vi "Populate Menu.vi"(8 "error in (no error)":errorcluster, 9 "Coords":T1, 10 "MenuRef":refnum<k9>, 11 "Test Executive View in":refnum<class "Test Executive View.lvclass">) -> (0 "error out":errorcluster, 2 "Discard?":bool, 3 "Test Executive View out":refnum<class "Test Executive View.lvclass">)   [LabVIEW 2019, in "Test Executive View.lvclass"]
uses:
  <vilib>/gpm_packages/@cs/Test-executive-builder/Example/Application/Test Executive View/Test Executive View/Test Executive View.lvclass
  C:/Program Files/National Instruments/LabVIEW 2019/vi.lib/gpm_packages/@cs/Test-executive-builder/Source/Test Executive Builder View/Test Executive Builder View/Test Executive Builder View.lvclass
  <vilib>/Utility/miscctls.llb/LVPoint32TypeDef.ctl
  <vilib>/gpm_packages/@cs/Test-executive-builder/Source/Test Executive Builder View/Test Executive Builder View/Test Executive Builder View.lvclass/Test Executive Builder View.ctl
  <vilib>/gpm_packages/@cs/Test-executive-builder/Source/Test Executive Builder View/Tree Click Interpreter/Tree Click Interpreter.lvclass
  <vilib>/gpm_packages/@cs/Test-executive-builder/Source/Test Executive Builder View/Test Executive Builder View/Test Executive Builder View.lvclass
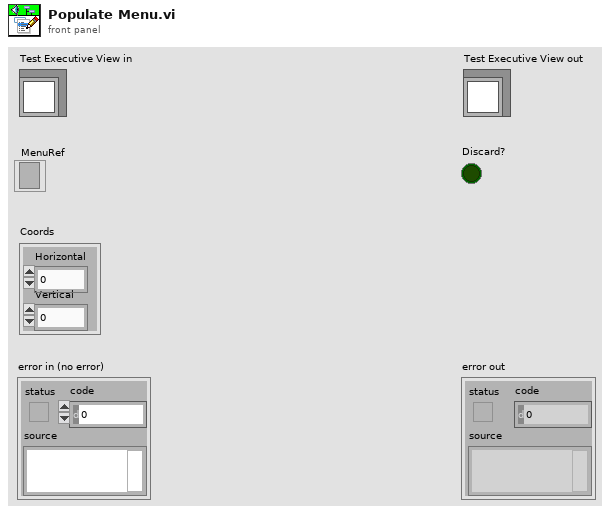
[diagram p1: front panel]
types:
  T1 = typedef "LVPoint32TypeDef.ctl" = cluster{"Horizontal":i32, "Vertical":i32}
  T2 = typedef "Relative Click Location.ctl" = enum16{"Unknown Location", "Below Element", "On Element", "Above Element"}
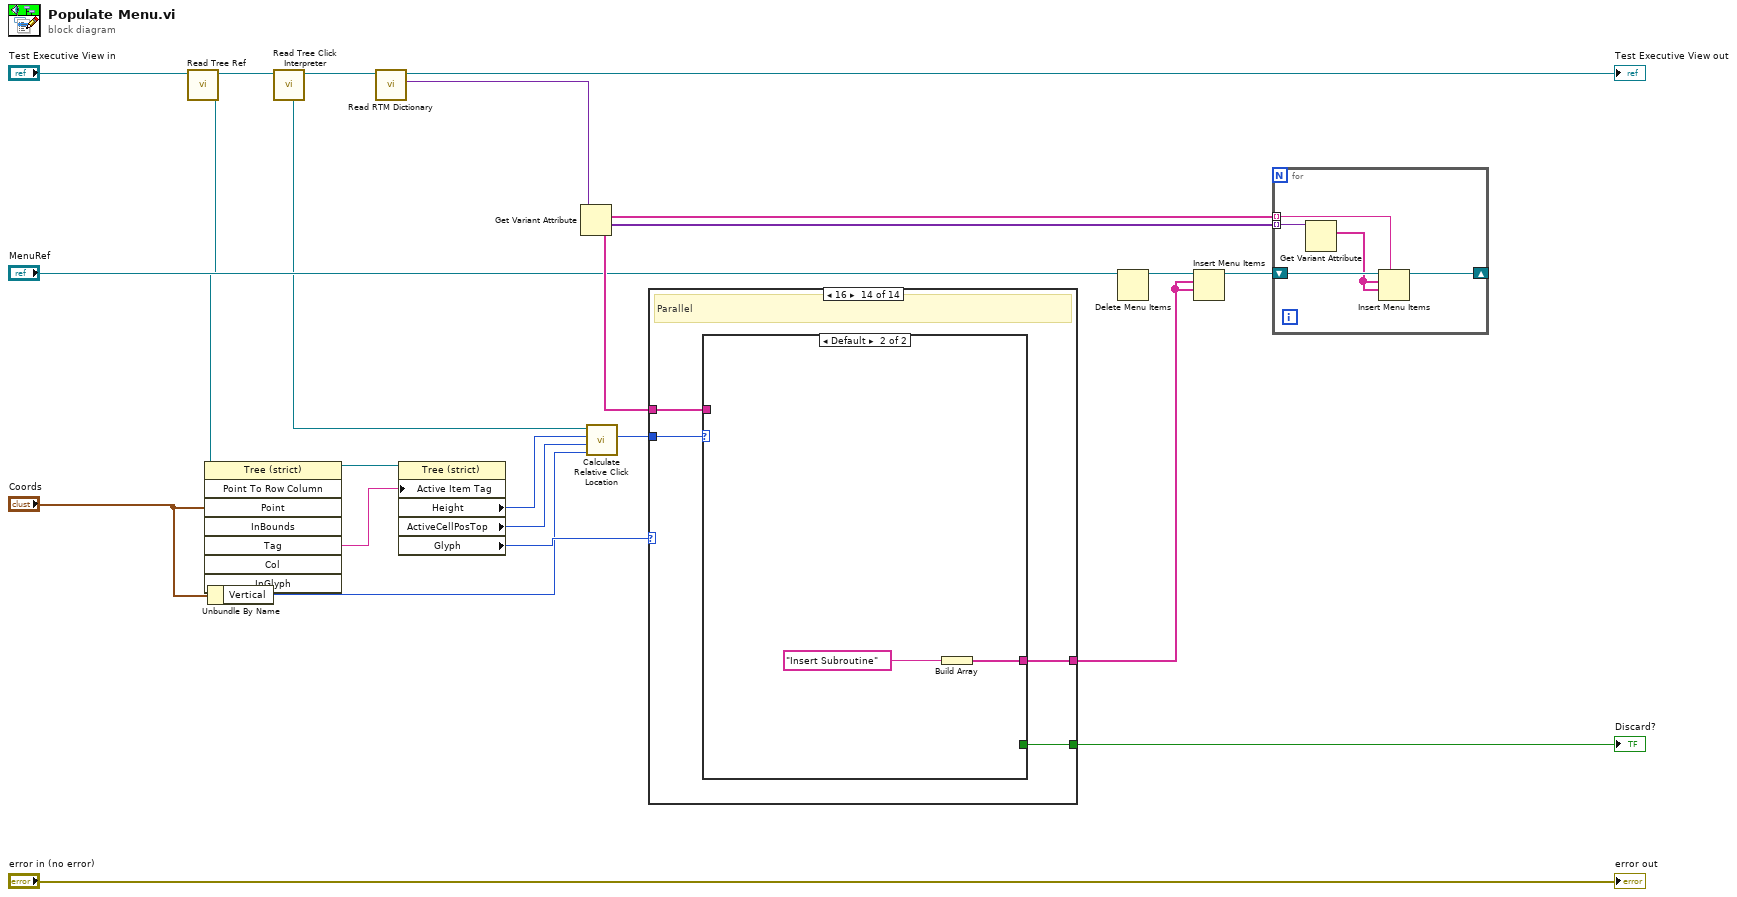
[diagram p0: block diagram]
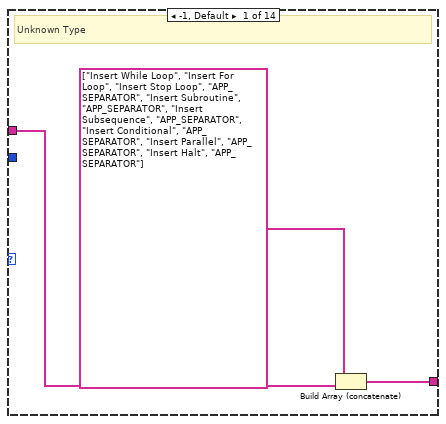
[diagram p2: hidden frame]
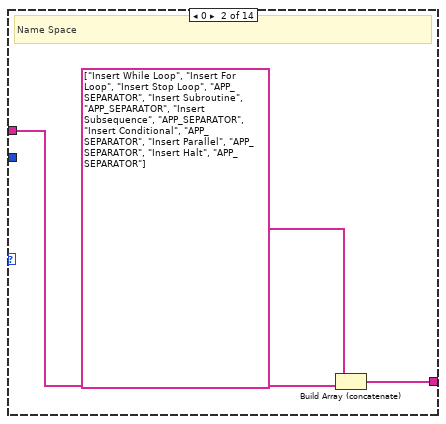
[diagram p3: hidden frame]
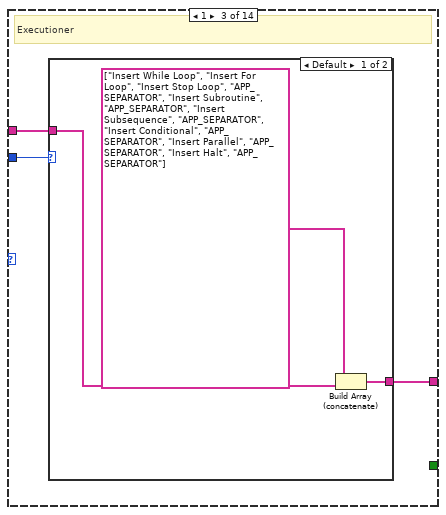
[diagram p4: hidden frame]
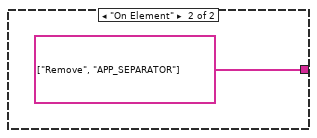
[diagram p5: hidden frame]
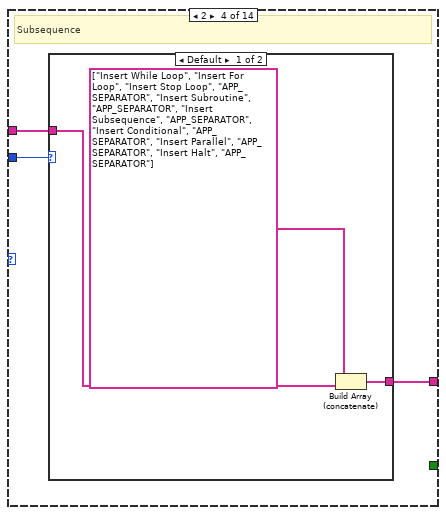
[diagram p6: hidden frame]
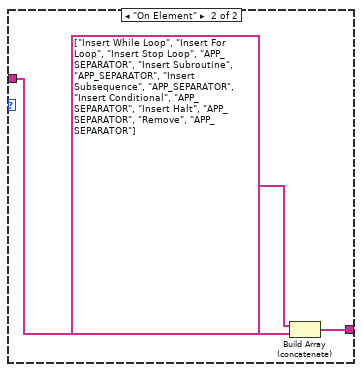
[diagram p7: hidden frame]
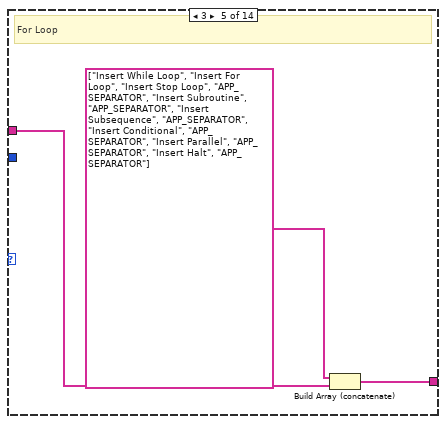
[diagram p8: hidden frame]
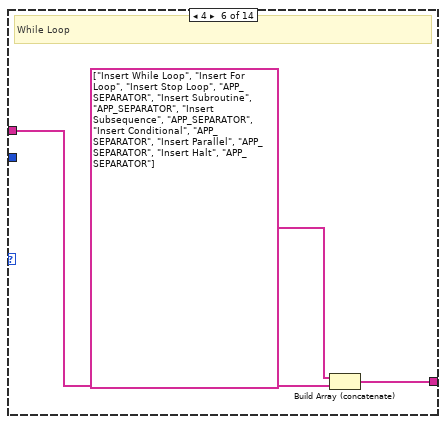
[diagram p9: hidden frame]
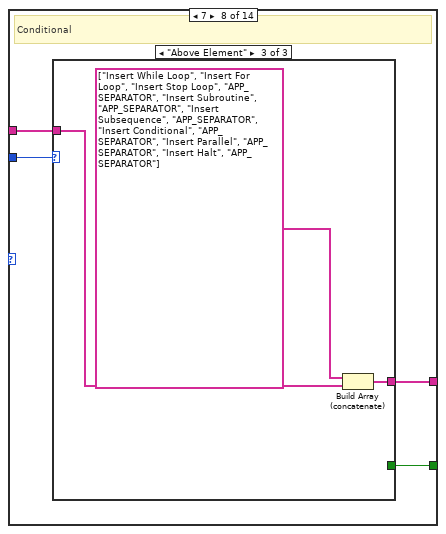
[diagram p11: hidden frame]
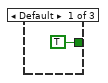
[diagram p12: hidden frame]
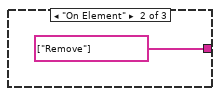
[diagram p13: hidden frame]
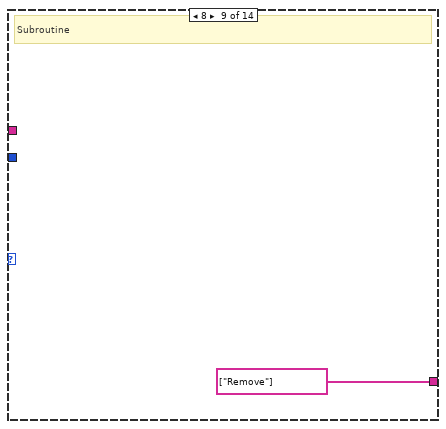
[diagram p14: hidden frame]
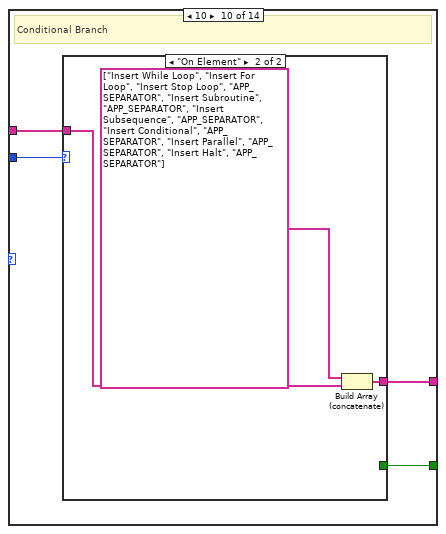
[diagram p15: hidden frame]
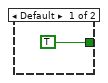
[diagram p16: hidden frame]
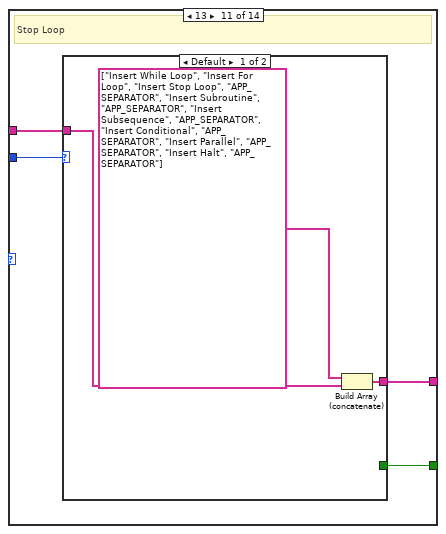
[diagram p17: hidden frame]
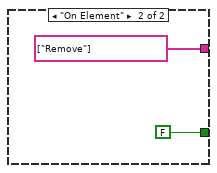
[diagram p18: hidden frame]
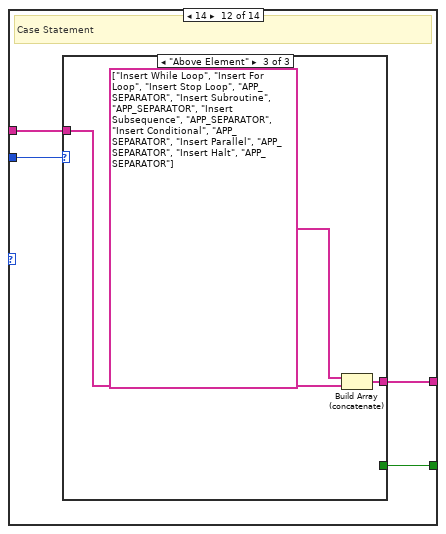
[diagram p19: hidden frame]
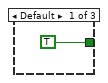
[diagram p20: hidden frame]
diagram:
  n1 = call <vilib>:"Read Tree Ref.vi"("Test Executive Builder View in"="Test Executive View in") -> ("Tree Ref"=w8:refnum<vi>, "Test Executive Builder View out"=w22:refnum<class "Test Executive View.lvclass">)  [unwired: 9 in]
  n2 = invoke class="Tree (strict)" method="Point To Row Column"(reference=w8, "Point"="Coords") -> (reference out=w16:refnum<vi>, "Tag"=w15:string)  [unwired: 6 in, 6 out]
  n3 = Unbundle By Name("Coords") -> ("Vertical"=w3:i32)
  n4 = call <vilib>:"Read Tree Click Interpreter.vi"("Test Executive Builder View in"=w22) -> ("Test Executive Builder View out"=w20:refnum<class "Test Executive View.lvclass">, "Tree Click Interpreter"=w6:refnum<class "Tree Click Interpreter.lvclass">)  [unwired: 9 in]
  n5 = call <vilib>:"Read RTM Dictionary.vi"("Test Executive Builder View in"=w20) -> ("RTM Dictionary"=w2:variant, "Test Executive Builder View out"=→"Test Executive View out":refnum<class "Test Executive View.lvclass">)  [unwired: 9 in]
  n6 = property class="Tree (strict)"(reference=w16, "Active Item Tag"=w15) -> ("Height"=w5:i32, "ActiveCellPosTop"=w4:i32, "Glyph"=w14:i32)  [unwired: 1 in, 2 out]
  n7 = Get Variant Attribute(Variant=w2) -> (names=w13:string[], values=w18:variant[])  [unwired: 3 in, 2 out]
  n8 = call-dynamic "Calculate Relative Click Location.vi"("Click Vertical Position"=w3, "Cell Top Position"=w4, "Cell Height"=w5, "Tree Click Interpreter in"=w6) -> ("Relative Click Location"=w7:T2)  [unwired: 6 in, 1 out]
  n9 = case shown="16" w14 {
    tunnel: w7 -> [_ _ w30 w37 _ _ _ w53 _ w65 w73 w82 w92 w101]
    tunnel: w13 -> [w25 w29 w32 w39 w48 w51 _ w52 _ w64 w72 w81 w91 w100]
    tunnel: [w24 w28 w31 w38 w47 w50 _ w54 string[] ["Remove"] w63 w71 w80 w90 w99] -> w12
    tunnel: [_ _ _ _ _ _ _ w55 _ w62 w70 w79 w89 w98] -> w1
    frame -1, Default {
      # "Unknown Type"
      n10 = Build Array (concatenate)(string[] ["Insert While Loop", "Insert For Loop", "Insert Stop Loop", "APP_SEPARATOR", "Insert Subroutine", "APP_SEPARATOR", "Insert Subsequence", "APP_SEPARATOR", "Insert Conditional", "APP_SEPARATOR", "Insert Parallel", "APP_SEPARATOR", "Insert Halt", "APP_SEPARATOR"], w25) -> (w24:string[])
    }
    frame 0 {
      # "Name Space"
      n11 = Build Array (concatenate)(string[] ["Insert While Loop", "Insert For Loop", "Insert Stop Loop", "APP_SEPARATOR", "Insert Subroutine", "APP_SEPARATOR", "Insert Subsequence", "APP_SEPARATOR", "Insert Conditional", "APP_SEPARATOR", "Insert Parallel", "APP_SEPARATOR", "Insert Halt", "APP_SEPARATOR"], w29) -> (w28:string[])
    }
    frame 1 {
      # "Executioner"
      n12 = case shown="Default" w30 {
        tunnel: w32 -> [w35 _]
        tunnel: [w34 string[] ["Remove", "APP_SEPARATOR"]] -> w31
        frame Default {
          n13 = Build Array (concatenate)(string[] ["Insert While Loop", "Insert For Loop", "Insert Stop Loop", "APP_SEPARATOR", "Insert Subroutine", "APP_SEPARATOR", "Insert Subsequence", "APP_SEPARATOR", "Insert Conditional", "APP_SEPARATOR", "Insert Parallel", "APP_SEPARATOR", "Insert Halt", "APP_SEPARATOR"], w35) -> (w34:string[])
        }
        frame "On Element" {
        }
      }
    }
    frame 2 {
      # "Subsequence"
      n14 = case shown="Default" w37 {
        tunnel: w39 -> [w42 w43]
        tunnel: [w41 w45] -> w38
        frame Default {
          n15 = Build Array (concatenate)(string[] ["Insert While Loop", "Insert For Loop", "Insert Stop Loop", "APP_SEPARATOR", "Insert Subroutine", "APP_SEPARATOR", "Insert Subsequence", "APP_SEPARATOR", "Insert Conditional", "APP_SEPARATOR", "Insert Parallel", "APP_SEPARATOR", "Insert Halt", "APP_SEPARATOR"], w42) -> (w41:string[])
        }
        frame "On Element" {
          n16 = Build Array (concatenate)(string[] ["Insert While Loop", "Insert For Loop", "Insert Stop Loop", "APP_SEPARATOR", "Insert Subroutine", "APP_SEPARATOR", "Insert Subsequence", "APP_SEPARATOR", "Insert Conditional", "APP_SEPARATOR", "Insert Halt", "APP_SEPARATOR", "Remove", "APP_SEPARATOR"], w43) -> (w45:string[])
        }
      }
    }
    frame 3 {
      # "For Loop"
      n17 = Build Array (concatenate)(string[] ["Insert While Loop", "Insert For Loop", "Insert Stop Loop", "APP_SEPARATOR", "Insert Subroutine", "APP_SEPARATOR", "Insert Subsequence", "APP_SEPARATOR", "Insert Conditional", "APP_SEPARATOR", "Insert Parallel", "APP_SEPARATOR", "Insert Halt", "APP_SEPARATOR"], w48) -> (w47:string[])
    }
    frame 4 {
      # "While Loop"
      n18 = Build Array (concatenate)(string[] ["Insert While Loop", "Insert For Loop", "Insert Stop Loop", "APP_SEPARATOR", "Insert Subroutine", "APP_SEPARATOR", "Insert Subsequence", "APP_SEPARATOR", "Insert Conditional", "APP_SEPARATOR", "Insert Parallel", "APP_SEPARATOR", "Insert Halt", "APP_SEPARATOR"], w51) -> (w50:string[])
    }
    frame 5 {
      # "Attribute"
    }
    frame 7 {
      # "Conditional"
      n19 = case shown="\"Above Element\"" w53 {
        tunnel: [TRUE _ _] -> w55
        tunnel: [_ string[] ["Remove"] w59] -> w54
        tunnel: w52 -> [_ _ w60]
        frame Default {
        }
        frame "On Element" {
        }
        frame "Above Element" {
          n20 = Build Array (concatenate)(string[] ["Insert While Loop", "Insert For Loop", "Insert Stop Loop", "APP_SEPARATOR", "Insert Subroutine", "APP_SEPARATOR", "Insert Subsequence", "APP_SEPARATOR", "Insert Conditional", "APP_SEPARATOR", "Insert Parallel", "APP_SEPARATOR", "Insert Halt", "APP_SEPARATOR"], w60) -> (w59:string[])
        }
      }
    }
    frame 8 {
      # "Subroutine"
    }
    frame 10 {
      # "Conditional Branch"
      n21 = case shown="\"On Element\"" w65 {
        tunnel: w64 -> [_ w69]
        tunnel: [_ w68] -> w63
        tunnel: [TRUE _] -> w62
        frame Default {
        }
        frame "On Element" {
          n22 = Build Array (concatenate)(string[] ["Insert While Loop", "Insert For Loop", "Insert Stop Loop", "APP_SEPARATOR", "Insert Subroutine", "APP_SEPARATOR", "Insert Subsequence", "APP_SEPARATOR", "Insert Conditional", "APP_SEPARATOR", "Insert Parallel", "APP_SEPARATOR", "Insert Halt", "APP_SEPARATOR"], w69) -> (w68:string[])
        }
      }
    }
    frame 13 {
      # "Stop Loop"
      n23 = case shown="Default" w73 {
        tunnel: w72 -> [w76 _]
        tunnel: [w75 string[] ["Remove"]] -> w71
        tunnel: [_ FALSE] -> w70
        frame Default {
          n24 = Build Array (concatenate)(string[] ["Insert While Loop", "Insert For Loop", "Insert Stop Loop", "APP_SEPARATOR", "Insert Subroutine", "APP_SEPARATOR", "Insert Subsequence", "APP_SEPARATOR", "Insert Conditional", "APP_SEPARATOR", "Insert Parallel", "APP_SEPARATOR", "Insert Halt", "APP_SEPARATOR"], w76) -> (w75:string[])
        }
        frame "On Element" {
        }
      }
    }
    frame 14 {
      # "Case Statement"
      n25 = case shown="\"Above Element\"" w82 {
        tunnel: w81 -> [_ _ w88]
        tunnel: [_ string[] ["Remove"] w87] -> w80
        tunnel: [TRUE FALSE _] -> w79
        frame Default {
        }
        frame "On Element" {
        }
        frame "Above Element" {
          n26 = Build Array (concatenate)(string[] ["Insert While Loop", "Insert For Loop", "Insert Stop Loop", "APP_SEPARATOR", "Insert Subroutine", "APP_SEPARATOR", "Insert Subsequence", "APP_SEPARATOR", "Insert Conditional", "APP_SEPARATOR", "Insert Parallel", "APP_SEPARATOR", "Insert Halt", "APP_SEPARATOR"], w88) -> (w87:string[])
        }
      }
    }
    frame 15 {
      # "Halt"
      n27 = case shown="\"On Element\"" w92 {
        tunnel: w91 -> [_ w97]
        tunnel: [string[] ["Remove"] w96] -> w90
        tunnel: [FALSE _] -> w89
        frame "On Element" {
        }
        frame Default {
          n28 = Build Array (concatenate)(string[] ["Insert While Loop", "Insert For Loop", "Insert Stop Loop", "APP_SEPARATOR", "Insert Subroutine", "APP_SEPARATOR", "Insert Subsequence", "APP_SEPARATOR", "Insert Conditional", "APP_SEPARATOR", "Insert Parallel", "APP_SEPARATOR", "Insert Halt", "APP_SEPARATOR"], w97) -> (w96:string[])
        }
      }
    }
    frame 16 {
      # "Parallel"
      n29 = case shown="Default" w101 {
        tunnel: w100 -> [_ _]
        tunnel: [string[] ["Remove"] w105] -> w99
        tunnel: [FALSE _] -> w98
        frame "On Element" {
        }
        frame Default {
          n30 = Build Array("Insert Subroutine") -> (w105:string[])
        }
      }
    }
  }
  "Discard?" <- w1
  n31 = Delete Menu Items(9:"MenuRef") -> (3:w19:refnum<k9>)  [unwired: 3 in, 1 out]
  n32 = Insert Menu Items(7:w12, 8:w12, 9:w19) -> (3:w17:refnum<k9>)  [unwired: 3 in, 2 out]
  n33 = for {
    tunnel: w13 -> [w107] mode=indexing
    tunnel: w18 -> [w110] mode=indexing
    shift-right: [w108] -> _
    shift-left: w17 -> [w109]
    n34 = Get Variant Attribute(Variant=w110) -> (names=w106:string[])  [unwired: 3 in, 3 out]
    n35 = Insert Menu Items(5:w107, 7:w106, 8:w106, 9:w109) -> (3:w108:refnum<k9>)  [unwired: 2 in, 2 out]
  }
  "error out" <- "error in (no error)"
